vi "Create ListBox.vi"(8 "Error In":errorcluster, 11 "Multicolumn Listbox Ref In":refnum<vi>) -> (0 "Error Out":errorcluster, 3 "Multicolumn Listbox Ref Out":refnum<vi>)   [LabVIEW 2017]
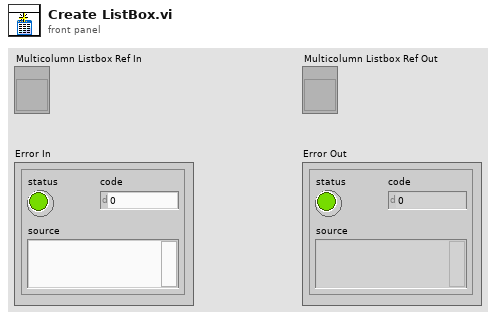
[diagram p1: front panel]
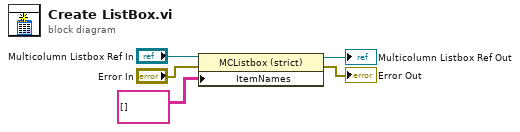
[diagram p0: block diagram]
diagram:
  n1 = property class="MCListbox (strict)"(reference="Multicolumn Listbox Ref In", error in="Error In", "ItemNames"=string[][] []) -> (reference out=→"Multicolumn Listbox Ref Out":refnum<vi>, error out=→"Error Out":errorcluster)
